vi "Stop Acquisition.vi"(8 "error in (no error)":errorcluster caption="错误输入（无错误）", 11 "Hardware Resources in":T1={"PLC设置"={"ActLogicalStationNumber"=0, "ActUtlType"=refnum}, "动作设置"={"自动跳法测试动作"={"夹紧"={"PLC指令"={"变量类型"=2, "PLC地址"=0, "size"=0, "写入数据(写入时有效)"=0}}, "通油"={"打开主阀"={"变量类型"=2, "PLC地址"=0, "size"=0, "写入数据(写入时有效)"=0}, "打开电磁阀"={"变量类型"=2, "PLC地址"=0, "size"=0, "写入数据(写入时有效)"=0}}, "压销"={"PLC指令"={"变量类型"=2, "PLC地址"=0, "size"=0, "写入数据(写入时有效)"=0}}}, "其他动作"={"其他指令1"={"变量类型"=2, "PLC地址"=0, "size"=0, "写入数据(写入时有效)"=0}, "其他指令2"={"变量类型"=2, "PLC地址"=0, "size"=0, "写入数据(写入时有效)"=0}, "其他指令3"={"变量类型"=2, "PLC地址"=0, "size"=0, "写入数据(写入时有效)"=0}, "其他指令4"={"变量类型"=2, "PLC地址"=0, "size"=0, "写入数据(写入时有效)"=0}, "其他指令5"={"变量类型"=2, "PLC地址"=0, "size"=0, "写入数据(写入时有效)"=0}}}, "电机设置"={"counter"="Dev1/ctr0", "方向端口"="", "当前方向"=FALSE, "频率"=0.0, "DAQmx Task"=""}, "所有测试电机转动逻辑"={"啮合测试电机转动逻辑"={"反转判断条件1"={"传感器序号"=0, "条件"=enum."小于", "值"=0.0, "条件判断时间间隔"=0, "反转等待时长"=0}, "停止判断条件1"={"角度传感器序号"=0, "正转/反转"=enum."正转", "反转次数"=0, "停止角度"=0.0, "停止角度误差范围"=0.0}}, "退回测试电机转动逻辑"={"反转判断条件1"={"传感器序号"=0, "条件"=enum."小于", "值"=0.0, "条件判断时间间隔"=0, "反转等待时长"=0}, "停止判断条件1"={"角度传感器序号"=0, "正转/反转"=enum."正转", "反转次数"=0, "停止角度"=0.0, "停止角度误差范围"=0.0}}, "功能测试电机转动逻辑"={"反转判断条件1"={"传感器序号"=0, "条件"=enum."小于", "值"=0.0, "条件判断时间间隔"=0, "反转等待时长"=0}, "停止判断条件1"={"角度传感器序号"=0, "正转/反转"=enum."正转", "反转次数"=0, "停止角度"=0.0, "停止角度误差范围"=0.0}}, "力特性测试电机转动逻辑"={"反转判断条件1"={"传感器序号"=0, "条件"=enum."小于", "值"=0.0, "条件判断时间间隔"=0, "反转等待时长"=0}, "停止判断条件1"={"角度传感器序号"=0, "正转/反转"=enum."正转", "反转次数"=0, "停止角度"=0.0, "停止角度误差范围"=0.0}}, "自动调阀测试分中电机转动逻辑"={"反转判断条件1"={"传感器序号"=0, "条件"=enum."小于", "值"=0.0, "条件判断时间间隔"=0, "反转等待时长"=0}, "停止判断条件1"={"角度传感器序号"=0, "正转/反转"=enum."正转", "反转次数"=0, "停止角度"=0.0, "停止角度误差范围"=0.0}}, "自动调阀测试对中电机转动逻辑"={"反转判断条件1"={"传感器序号"=0, "条件"=enum."小于", "值"=0.0, "条件判断时间间隔"=0, "反转等待时长"=0}, "停止判断条件1"={"角度传感器序号"=0, "正转/反转"=enum."正转", "反转次数"=0, "停止角度"=0.0, "停止角度误差范围"=0.0}}}} caption="硬件资源输入" {"动作设置"."其他动作"."其他指令5"."变量类型" items=["X", "Y", "M", "D"]; "动作设置"."其他动作"."其他指令4"."变量类型" items=["X", "Y", "M", "D"]; "动作设置"."其他动作"."其他指令3"."变量类型" items=["X", "Y", "M", "D"]; "动作设置"."其他动作"."其他指令2"."变量类型" items=["X", "Y", "M", "D"]; "动作设置"."其他动作"."其他指令1"."变量类型" items=["X", "Y", "M", "D"]; "动作设置"."自动跳法测试动作"."压销"."PLC指令"."变量类型" items=["X", "Y", "M", "D"]; "动作设置"."自动跳法测试动作"."通油"."打开电磁阀"."变量类型" items=["X", "Y", "M", "D"]; "动作设置"."自动跳法测试动作"."通油"."打开主阀"."变量类型" items=["X", "Y", "M", "D"]; "动作设置"."自动跳法测试动作"."夹紧"."PLC指令"."变量类型" items=["X", "Y", "M", "D"]}) -> (0 "error out":errorcluster caption="错误输出")   [LabVIEW 2015, in "Action.lvlib"]
doc: "停止采集。"
uses:
  Action.lvlib
  Hardware Configuration.ctl
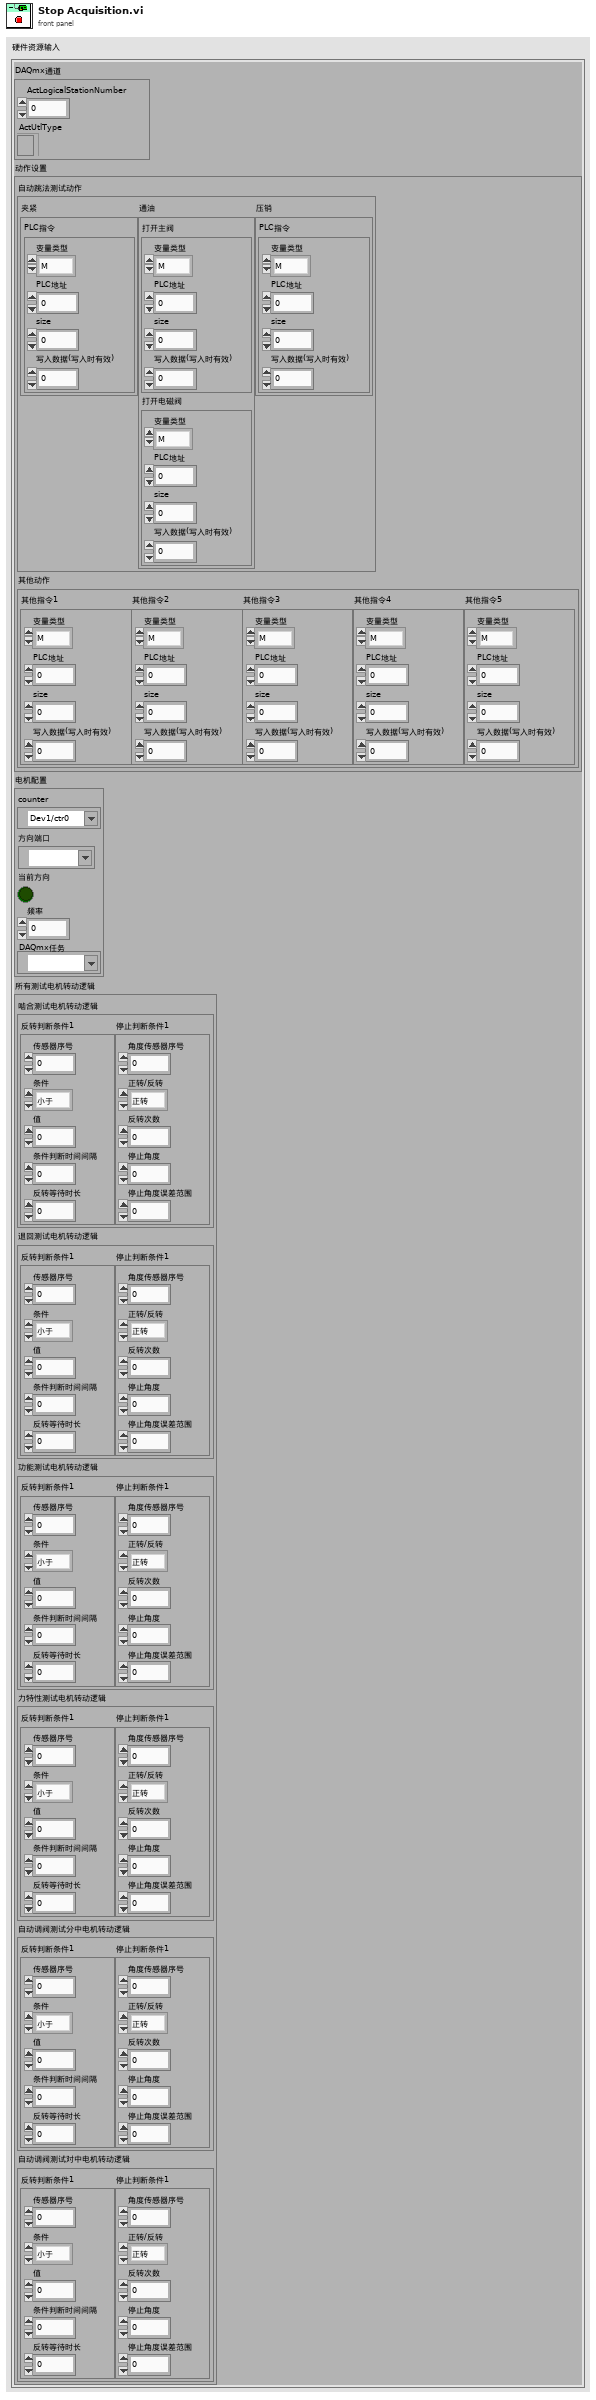
[diagram p1: front panel]
types:
  T1 = typedef "Action.lvlib/Hardware Configuration.ctl" = cluster{"PLC设置":T2, "动作设置":T3, "电机设置":T7, "所有测试电机转动逻辑":T8}
  T2 = typedef "Action.lvlib/PLC设置.ctl" = cluster{"ActLogicalStationNumber":i32, "ActUtlType":refnum<k7>}
  T3 = typedef "Action.lvlib/动作设置.ctl" = cluster{"自动跳法测试动作":T4, "其他动作":T6}
  T4 = typedef "Action.lvlib/自动调阀测试动作设置.ctl" = cluster{"夹紧":cluster{"PLC指令":T5}, "通油":cluster{"打开主阀":T5, "打开电磁阀":T5}, "压销":cluster{"PLC指令":T5}}
  T5 = typedef "Action.lvlib/PLC控制指令.ctl" = cluster{"变量类型":u32, "PLC地址":i32, "size":i32, "写入数据(写入时有效)":i16}
  T6 = typedef "Action.lvlib/其他动作设置 .ctl" = cluster{"其他指令1":T5, "其他指令2":T5, "其他指令3":T5, "其他指令4":T5, "其他指令5":T5}
  T7 = typedef "Action.lvlib/电机控制设置.ctl" = cluster{"counter":tag, "方向端口":tag, "当前方向":bool, "频率":dbl, "DAQmx Task":refnum<k21>}
  T8 = typedef "Action.lvlib/所有测试电机转动逻辑.ctl" = cluster{"啮合测试电机转动逻辑":T9, "退回测试电机转动逻辑":T9, "功能测试电机转动逻辑":T9, "力特性测试电机转动逻辑":T9, "自动调阀测试分中电机转动逻辑":T9, "自动调阀测试对中电机转动逻辑":T9}
  T9 = typedef "Action.lvlib/电机转动逻辑1.ctl" = cluster{"反转判断条件1":T10, "停止判断条件1":T11}
  T10 = typedef "Action.lvlib/反转判断条件1.ctl" = cluster{"传感器序号":i32, "条件":enum16{"小于", "大于", "等于"}, "值":dbl, "条件判断时间间隔":i32, "反转等待时长":i32}
  T11 = typedef "Action.lvlib/停止判断条件1.ctl" = cluster{"角度传感器序号":i32, "正转/反转":enum16{"正转", "反转"}, "反转次数":i32, "停止角度":dbl, "停止角度误差范围":dbl}
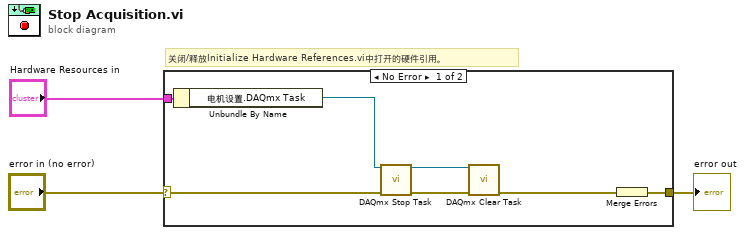
[diagram p0: block diagram]
diagram:
  # "关闭/释放Initialize Hardware References.vi中打开的硬件引用。"
  n1 = case shown="No Error" "error in (no error)" {
    selector: "error in (no error)" -> [w8 w11]
    tunnel: [w10 w11] -> w2
    tunnel: "Hardware Resources in" -> [w9 _]
    frame No Error {
      n2 = Unbundle By Name(w9) -> ("电机设置.DAQmx Task"=w7:refnum<k21>)
      n3 = call <vilib>:"DAQmx Stop Task.vi"("task/channels in"=w7, "error in"=w8) -> ("task out"=w6:refnum<k21>, "error out"=w5:errorcluster)  [unwired: 12 in]
      n4 = call <vilib>:"DAQmx Clear Task.vi"("task in"=w6, "error in"=w5) -> ("error out"=w4:errorcluster)  [unwired: 13 in]
      n5 = Merge Errors(w4) -> (w10:errorcluster)
    }
    frame Error {
    }
  }
  "error out" <- w2
